vi "Line Configuration Dialog.vi"(8 "error in":errorcluster, 9 "engine configuration in":refnum<class "engine configuration.lvclass">, 10 "tag bus configurable plugin module configuration":refnum<class "FPGA Module configuration.lvclass">, 11 "Line":T3) -> (0 "error out":errorcluster, 1 "success":bool, 2 "changed":bool, 3 "Mappings out":T2)   [LabVIEW 2017, in "FPGA Module editor node.lvclass"]
doc: "A dialog for allowing a user to specify the values of a new line."
uses:
  FPGA Module editor node.lvclass
  module/configuration/Line.ctl
  <vilib>/NI/Tag Bus Module Framework/channel/TBM channel.lvclass
  fpga channel/FPGA Channel.lvclass
  C:/Program Files (x86)/National Instruments/LabVIEW 2017/vi.lib/NI/Tag Bus Module Framework/channel/TBM channel.lvclass
  C:/Program Files (x86)/National Instruments/LabVIEW 2017/vi.lib/NI/Tag Bus/tag/tag descriptor.lvclass
  Mappings.ctl
  Map.ctl
  permissions.ctl
  <vilib>/NI/Module Execution Interface/Engine Configuration/engine configuration.lvclass
  module/configuration/FPGA Module configuration.lvclass
  C:/Program Files (x86)/National Instruments/LabVIEW 2017/vi.lib/NI/Configuration Framework/serializable configuration/NISE_CEF_serializable configuration.lvclass
  <vilib>/NI/Tag Bus Module Framework/channel/TBM channel.lvclass/TBM channel.ctl
  <vilib>/NI/Tag Bus/tag/tag descriptor.lvclass/tag descriptor.ctl
  <vilib>/NI/Configuration Framework/serializable configuration/NISE_CEF_serializable configuration.lvclass/NISE_CEF_serializable configuration.ctl
  <vilib>/NI/Tag Bus/tag/write tag name.vi
  <vilib>/NI/Tag Bus/tag/write data type.vi
  <vilib>/NI/Tag Bus Module Framework/channel/Write channel classification.vi
  <vilib>/NI/Configuration Framework/serializable configuration/Read UID.vi
  <vilib>/NI/Tag Bus Module Framework/channel/Read channel classification.vi
  <vilib>/NI/Tag Bus/tag/read data type.vi
  <vilib>/Utility/LVClass/Get LV Class Name.vi
  <vilib>/NI/Configuration Framework/error generator/NISE_error generator.vi
  <vilib>/NI/Tag Bus/tag/tag descriptor.lvclass
  <vilib>/NI/DCAF UI Toolkit/Controls/DCAF UI Elements.lvlib
panel:
  out "errors":string
  in  "Access Type":T1
  in  "Tag":i32(listbox)
  in  "Data Type":i32(listbox)
  in  "Channel Name":string
  in  "cancel":bool
  in  "ok":bool
  # "#CodeRecommended Add implementation details here. For example, a shared variable URL."
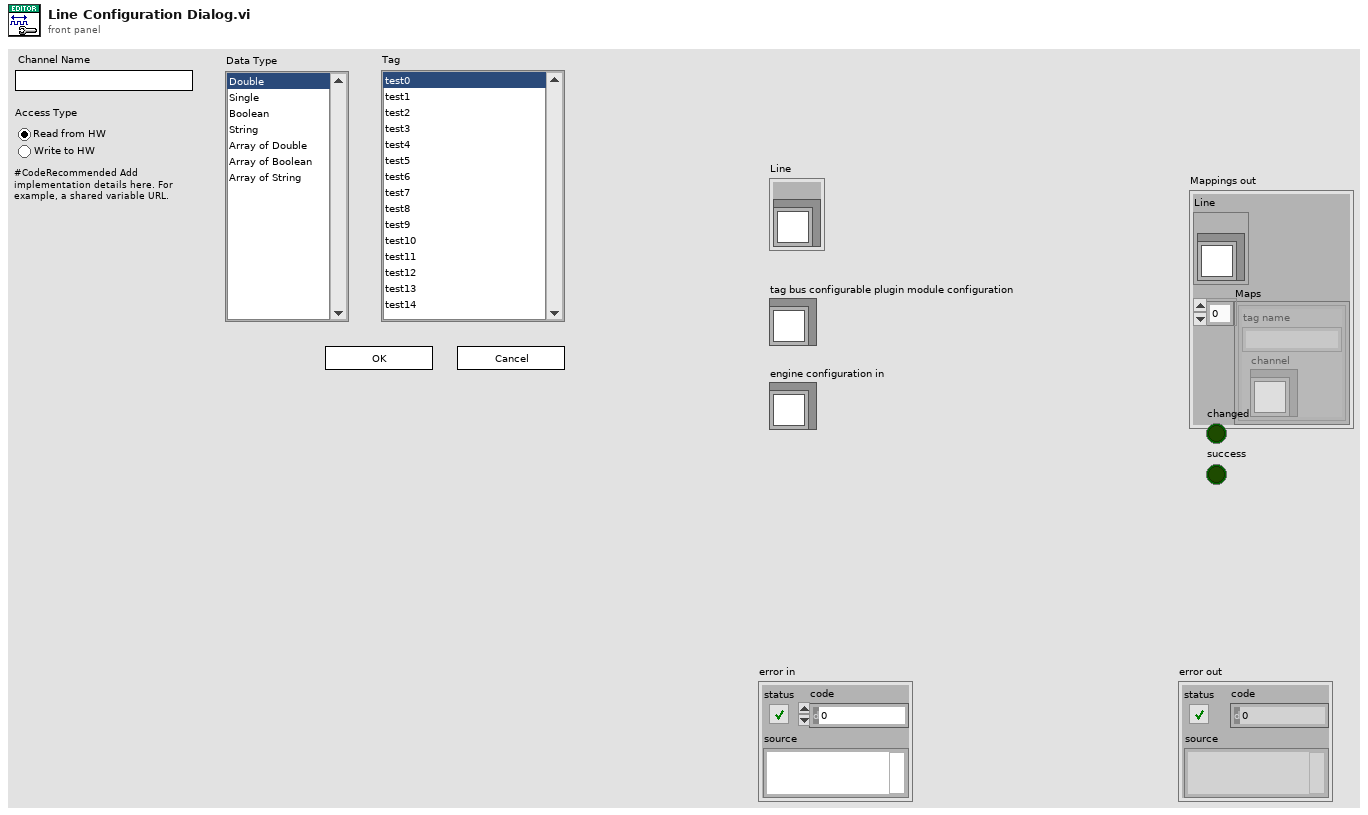
[diagram p1: front panel]
types:
  T1 = typedef "FPGA Module editor node.lvclass/permissions.ctl" = enum32{"Read from HW", "Write to HW"}
  T2 = typedef "FPGA Module editor node.lvclass/Mappings.ctl" = cluster{"Line":T3, "Maps":T4[]}
  T3 = typedef "FPGA Module configuration.lvclass/Line.ctl" = cluster{"Channel":refnum<class "FPGA Channel.lvclass">}
  T4 = typedef "FPGA Module editor node.lvclass/Map.ctl" = cluster{"channel":refnum<class "TBM channel.lvclass">, "tag name":string}
  T5 = typedef "tag bus.lvlib/tag descriptor.lvclass/Data Type.ctl" = enum16{"Double", "Single", "I64", "I32", "I16", "I8", "U64", "U32", "U16", "U8", "Boolean", "String", "Array of Double", "Array of Single", "Array of I64", "Array of I32", "Array of I16", "Array of I8", "Array of U64", "Array of U32", "Array of U16", "Array of U8", "Array of Boolean", "Array of String"}
  T6 = typedef "TBM channel.lvclass/channel classification.ctl" = enum16{"input data", "output data", "processing parameter", "processing result"}
  T7 = enum8{"Enabled", "Disabled", "Disabled and Grayed Out"}
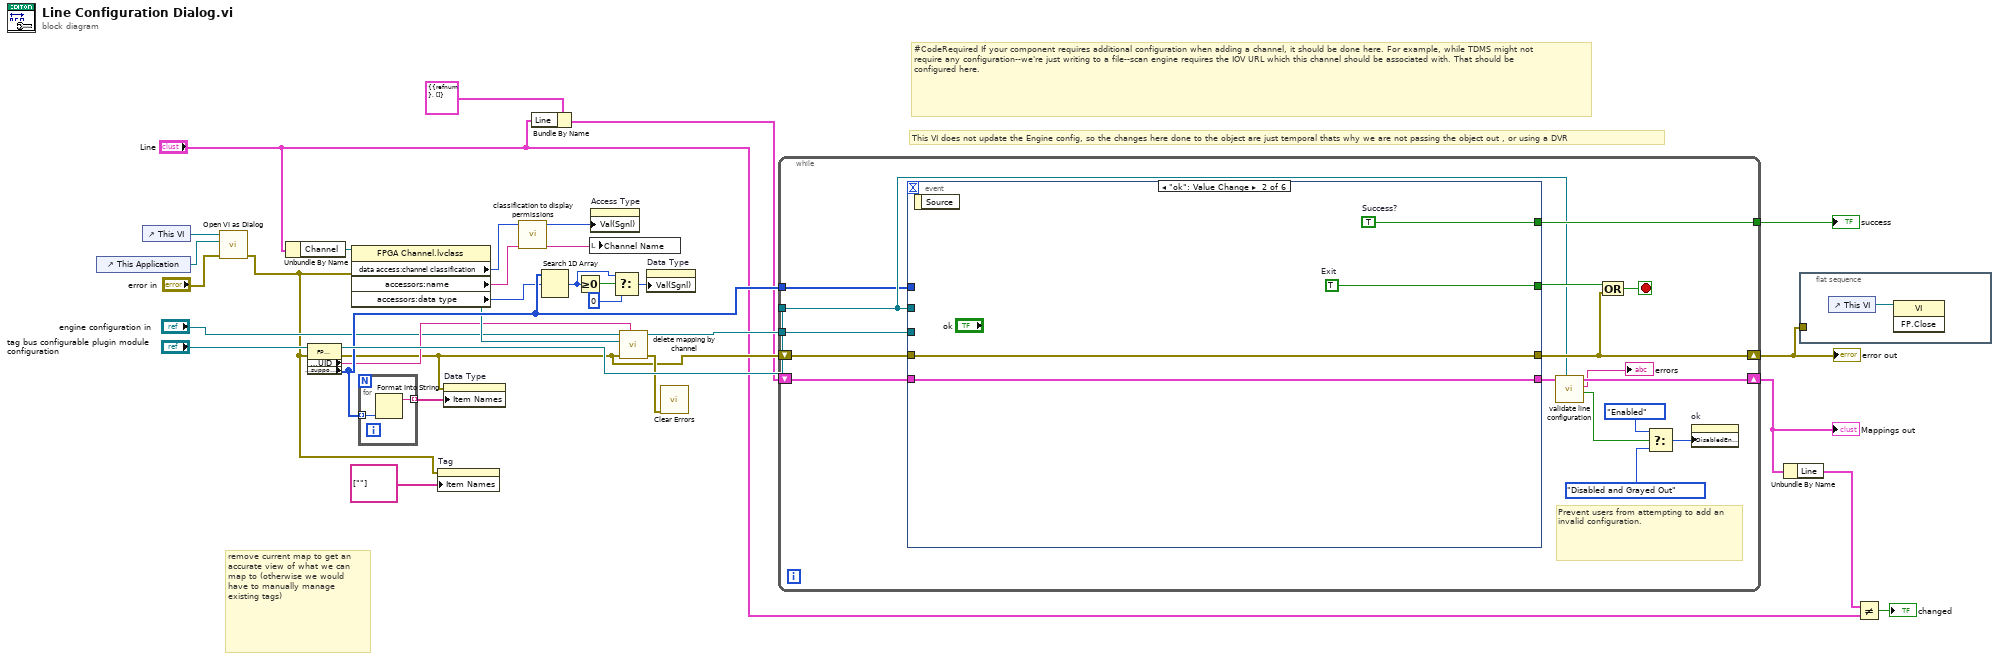
[diagram p0: block diagram]
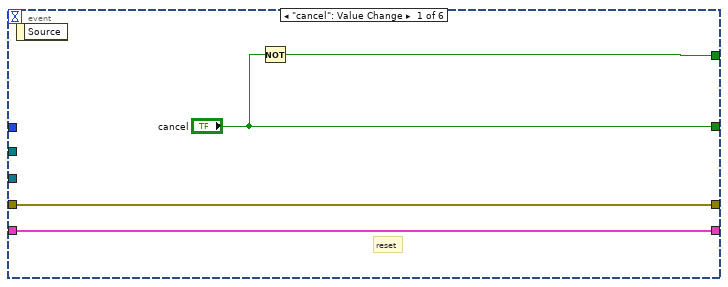
[diagram p2: hidden frame]
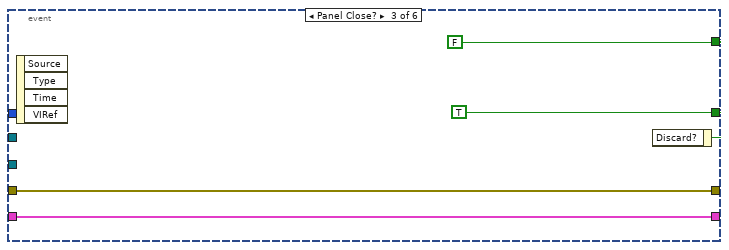
[diagram p3: hidden frame]
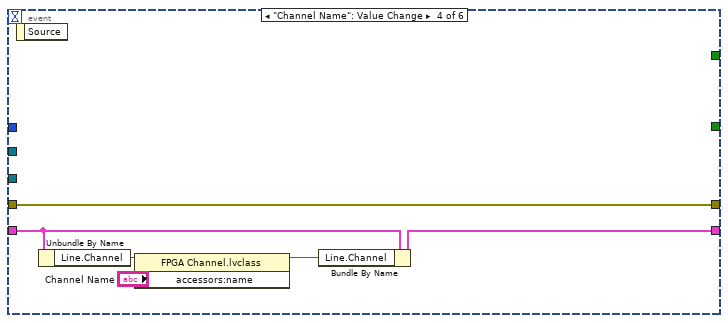
[diagram p4: hidden frame]
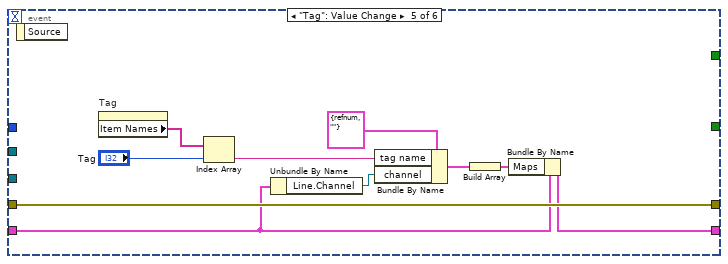
[diagram p5: hidden frame]
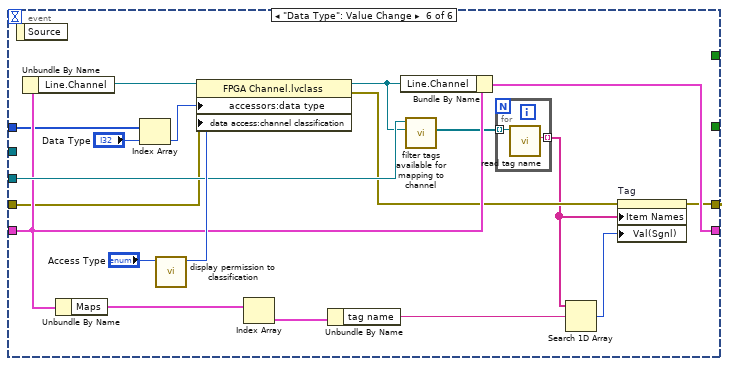
[diagram p6: hidden frame]
diagram:
  # "This VI does not update the Engine config, so the changes here done to the object are just temporal thats why we are not passing the object out , or using a DVR"
  # "remove current map to get an accurate view of what we can map to (otherwise we would have to manually manage existing tags)"
  # "#CodeRequired If your component requires additional configuration when adding a channel, it should be done here. For example, while TDMS might not require any configuration--we're just writing to a file--scan engine requires the IOV URL which this channel should be associated with. That should be configured here."
  n1 = control-ref of="This Application"() -> (w3:refnum<vi>)
  n2 = control-ref of="This VI"() -> (w4:refnum<vi>)
  n3 = call <vilib>:"Open VI as Dialog.vi"("error in (no error)"="error in", "This Application"=w3, "VI in"=w4) -> ("error out"=w1:errorcluster)  [unwired: 8 in]
  n4 = Unbundle By Name("Line") -> ("Channel"=w24:refnum<class "FPGA Channel.lvclass">)
  n5 = property class="FPGA Module configuration"(reference="tag bus configurable plugin module configuration", error in=w1) -> (reference out=w29:refnum<class "FPGA Module configuration.lvclass">, error out=w11:errorcluster, "Properties:UID"=w22:string, "Customize:Properties:supported types"=w28:T5[])
  n6 = property class="FPGA Channel.lvclass"(reference=w24, error in=w1) -> (reference out=w23:refnum<class "FPGA Channel.lvclass">, "data access:channel classification"=w26:T6, "accessors:name"=w25:string, "accessors:data type"=w14:T5)  [unwired: 1 out]
  n7 = for {
    tunnel: w28 -> [w34] mode=indexing
    tunnel: [w33] -> w21 mode=indexing
    n8 = Format Into String(w34) -> (resulting string=w33:string)  [unwired: 3 in, 1 out]
  }
  n9 = property on="Tag" class="LstBox (strict)"(error in=w1, "Item Names"=string[] [""]) -> ()  [unwired: 1 in, 2 out]
  n10 = property on="Data Type" class="LstBox (strict)"(error in=w11, "Item Names"=w21) -> ()  [unwired: 1 in, 2 out]
  n11 = call "classification to display permissions.vi"("channel classification"=w26) -> ("permissions"=w15:T1)  [unwired: 10 in]
  n12 = Bundle By Name(cluster=T2 {"Line"={"Channel"=refnum}, "Maps"=[]} ("Mappings out"), "Line"="Line") -> (w7:T2)
  n13 = Search 1D Array(1D array=w28, element=w14) -> (index of element=w19:i32)  [unwired: 1 in]
  n14 = Greater Or Equal To 0?(x=w19) -> (x >= 0?=w20:bool)
  n15 = local write "Channel Name"(w25) -> ()
  n16 = property on="Access Type" class="RadioBtnsControl (strict)"("Val(Sgnl)"=w15) -> ()  [unwired: 2 in, 2 out]
  n17 = Select(t=w19, s=w20, f=0) -> (s? t:f=w17:i32)
  n18 = call <vilib>:"delete mapping by channel.vi"("owner ID"=w22, "error in"=w11, "channel"=w23, "engine configuration in"="engine configuration in") -> ("error out"=w13:errorcluster, "engine configuration out"=w30:refnum<class "engine configuration.lvclass">)  [unwired: 6 in]
  n19 = property on="Data Type" class="LstBox (strict)"("Val(Sgnl)"=w17) -> ()  [unwired: 2 in, 2 out]
  n20 = call <vilib>:"Clear Errors.vi"("error in (no error)"=w13) -> ()  [unwired: 5 in, 2 out]
  n21 = while {
    shift-right: [w42] -> w27
    shift-left: w11 -> [w49]
    tunnel: [w48] -> w32
    shift-right: [w43] -> w5
    shift-left: w7 -> [w45]
    tunnel: w30 -> [w50]
    tunnel: w29 -> [w37]
    tunnel: w28 -> [w36]
    stop <- w46 stop-if-true
    # "Prevent users from attempting to add an invalid configuration."
    n22 = event shown="[1] \"ok\": Value Change" {
      selector: _ -> [_ _ _ _ _ _]
      dyn-events: _ -> [_ _ _ _ _ _]
      timeout: _ -> [_ _ _ _ _ _]
      tunnel: w50 -> [_ _ _ _ _ w95]
      tunnel: w49 -> [w54 w58 w62 w68 w78 w89]
      tunnel: [w54 w58 w62 w68 w78 w84] -> w42
      tunnel: [w53 w55 FALSE _ _ _] -> w48
      tunnel: ["cancel" w56 w60 _ _ _] -> w47
      tunnel: w45 -> [w51 w57 w59 w66 w72 w93]
      tunnel: [w51 w57 w59 w67 w69 w92] -> w44
      tunnel: w37 -> [_ _ _ _ _ _]
      tunnel: w36 -> [_ _ _ _ _ w88]
      event "cancel": Value Change {
        # "reset"
        n23 = event-data() -> ()  [unwired: 1 in, 1 out]
        n24 = Not(x="cancel") -> (.not. x?=w53:bool)
      }
      event "ok": Value Change {
        w55 = TRUE  # Success?
        w56 = TRUE  # Exit
        n25 = event-data() -> ()  [unwired: 1 in, 1 out]
      }
      event Panel Close? {
        w60 = TRUE ("cancel")
        n26 = event-data() -> ()  [unwired: 1 in, 4 out]
        n27 = event-data("Discard?"=w60) -> ()  [unwired: 1 in, 1 out]
      }
      event "Channel Name": Value Change {
        n28 = event-data() -> ()  [unwired: 1 in, 1 out]
        n29 = Unbundle By Name(w66) -> ("Line.Channel"=w65:refnum<class "FPGA Channel.lvclass">)
        n30 = property class="FPGA Channel.lvclass"(reference=w65, "accessors:name"="Channel Name") -> (reference out=w64:refnum<class "FPGA Channel.lvclass">)  [unwired: 1 in, 1 out]
        n31 = Bundle By Name(cluster=w66, "Line.Channel"=w64) -> (w67:T2)
      }
      event "Tag": Value Change {
        n32 = event-data() -> ()  [unwired: 1 in, 1 out]
        n33 = property on="Tag" class="LstBox (strict)"() -> ("Item Names"=w76:string[])  [unwired: 2 in, 2 out]
        n34 = Index Array(array=w76, index="Tag") -> (element=w75:string)
        n35 = Unbundle By Name(w72) -> ("Line.Channel"=w73:refnum<class "FPGA Channel.lvclass">)
        n36 = Bundle By Name(cluster=T4 {"channel"=refnum, "tag name"=""} ("Map"), "tag name"=w75, "channel"=w73) -> (w71:T4)
        n37 = Build Array(w71) -> (w70:T4[])
        n38 = Bundle By Name(cluster=w72, "Maps"=w70) -> (w69:T2)
      }
      event "Data Type": Value Change {
        n39 = event-data() -> ()  [unwired: 1 in, 1 out]
        n40 = Unbundle By Name(w93) -> ("Line.Channel"=w97:refnum<class "FPGA Channel.lvclass">)
        n41 = Unbundle By Name(w93) -> ("Maps"=w81:T4[])
        n42 = Index Array(array=w88, index="Data Type") -> (element=w86:T5)
        n43 = call "display permission to classification.vi"("display permissions"="Access Type") -> ("channel classification"=w96:T6)  [unwired: 10 in]
        n44 = property class="FPGA Channel.lvclass"(reference=w97, error in=w89, "accessors:data type"=w86, "data access:channel classification"=w96) -> (reference out=w94:refnum<class "FPGA Channel.lvclass">, error out=w85:errorcluster)
        n45 = Index Array(array=w81) -> (element=w80:T4)  [unwired: 1 in]
        n46 = Unbundle By Name(w80) -> ("tag name"=w79:string)
        n47 = Bundle By Name(cluster=w93, "Line.Channel"=w94) -> (w92:T2)
        n48 = call-dynamic "filter tags available for mapping to channel.vi"("channel to map to"=w94, "engine configuration in"=w95) -> ("filtered tags"=w91:refnum<class "tag descriptor.lvclass">[])  [unwired: 8 in, 1 out]
        n49 = for {
          tunnel: w91 -> [w99] mode=indexing
          tunnel: [w98] -> w83 mode=indexing
          n50 = call <vilib>:"read tag name.vi"("system tag in"=w99) -> ("name"=w98:string)  [unwired: 8 in, 2 out]
        }
        n51 = Search 1D Array(1D array=w83, element=w79) -> (index of element=w82:i32)  [unwired: 1 in]
        n52 = property on="Tag" class="LstBox (strict)"(error in=w85, "Item Names"=w83, "Val(Sgnl)"=w82) -> (error out=w84:errorcluster)  [unwired: 1 in, 1 out]
      }
    }
    n53 = call "validate line configuration.vi"("Module Config"=w37, "Mappings in"=w44) -> ("valid?"=w41:bool, "errors"=→"errors":string, "Mappings out"=w43:T2)  [unwired: 7 in]
    n54 = Compound Arithmetic op=OR(w47, w42) -> (w46:bool)
    n55 = Select(t=T7."Enabled" ("Disabled"), s=w41, f=T7."Disabled and Grayed Out") -> (s? t:f=w38:T7)
    n56 = property on="ok" class="Bool"("DisabledEnum"=w38) -> ()  [unwired: 2 in, 2 out]
  }
  "error out" <- w27
  "success" <- w32
  "Mappings out" <- w5
  n57 = Unbundle By Name(w5) -> ("Line"=w6:T3)
  n58 = flat-sequence {
    tunnel: w27 -> [_]
    frame #0 {
      n59 = control-ref of="This VI"() -> (w100:refnum<vi>)
      n60 = invoke class="VI" method="FP.Close"(reference=w100) -> ()  [unwired: 2 in, 3 out]
    }
  }
  n61 = Not Equal?(x=w6, y="Line") -> (x != y?=→"changed":bool)
